vi "Determine More Warnings.vi"(6 "Vitesse max. du vent":dbl, 7 "Vitesse actuelle du vent":dbl, 8 "entrée d'erreur (pas d'erreur)":errorcluster, 9 "Temp. min.":dbl, 10 "Temp. max.":dbl, 11 "Temp. actuelle":dbl) -> (0 "sortie d'erreur":errorcluster, 1 "Mise en garde ?":bool, 2 "Texte de mise en garde":string)   [LabVIEW 2009]
uses:
  Det Warnings.ctl
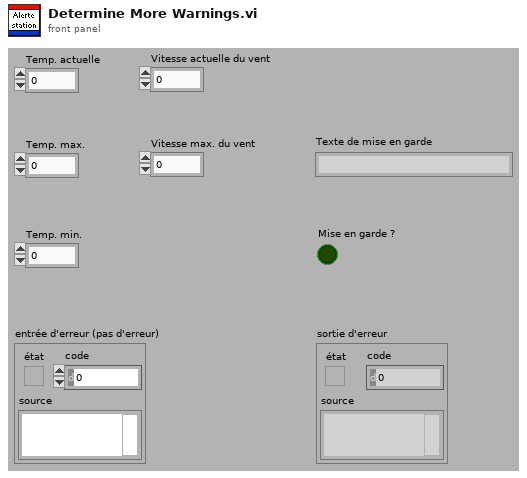
[diagram p1: front panel]
types:
  T1 = typedef "Det Warnings.ctl" = enum16{"Canicule", "Gel", "Vent fort", "Générer une msie en garde", "Détection d'erreur"}
  T2 = cluster{"Temp. actuelle":dbl, "Temp. max.":dbl, "Temp. min.":dbl, "Vitesse actuelle du vent":dbl, "Vitesse max. du vent":dbl}
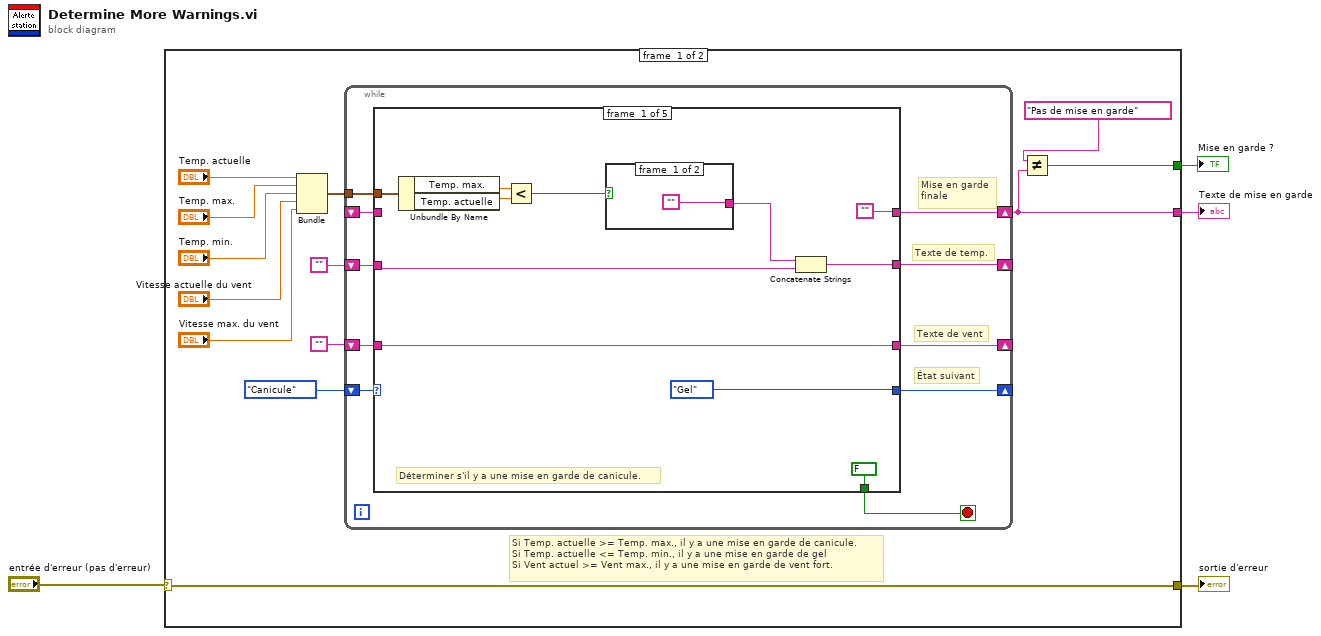
[diagram p0: block diagram]
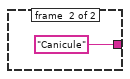
[diagram p2: hidden frame]
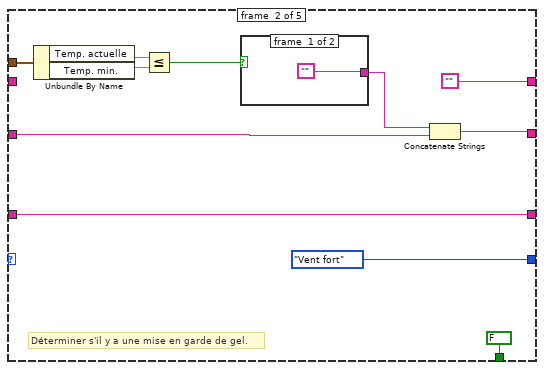
[diagram p3: hidden frame]
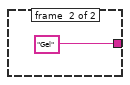
[diagram p4: hidden frame]
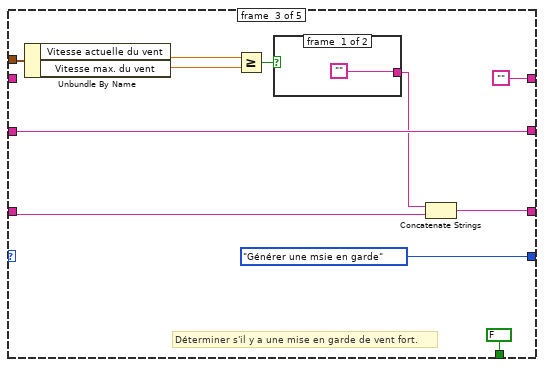
[diagram p5: hidden frame]
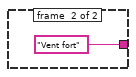
[diagram p6: hidden frame]
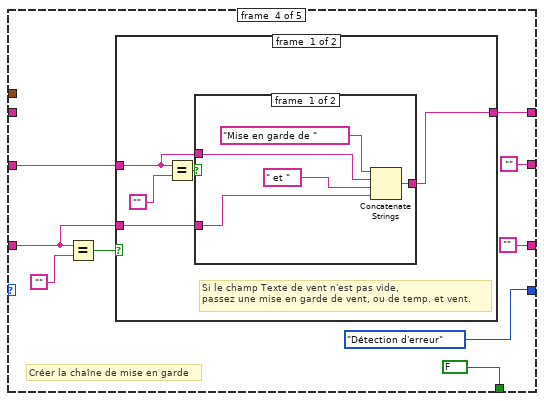
[diagram p7: hidden frame]
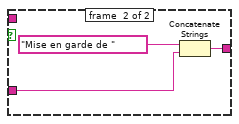
[diagram p8: hidden frame]
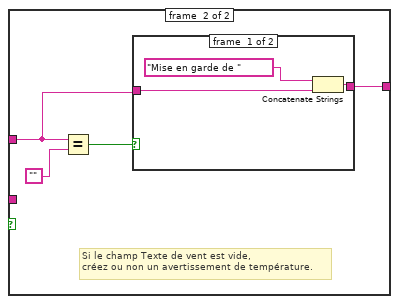
[diagram p9: hidden frame]
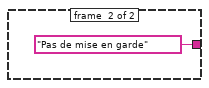
[diagram p10: hidden frame]
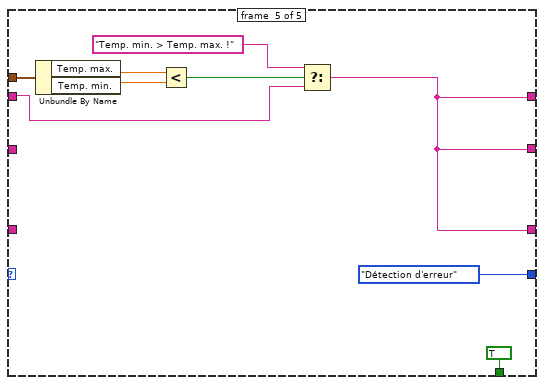
[diagram p11: hidden frame]
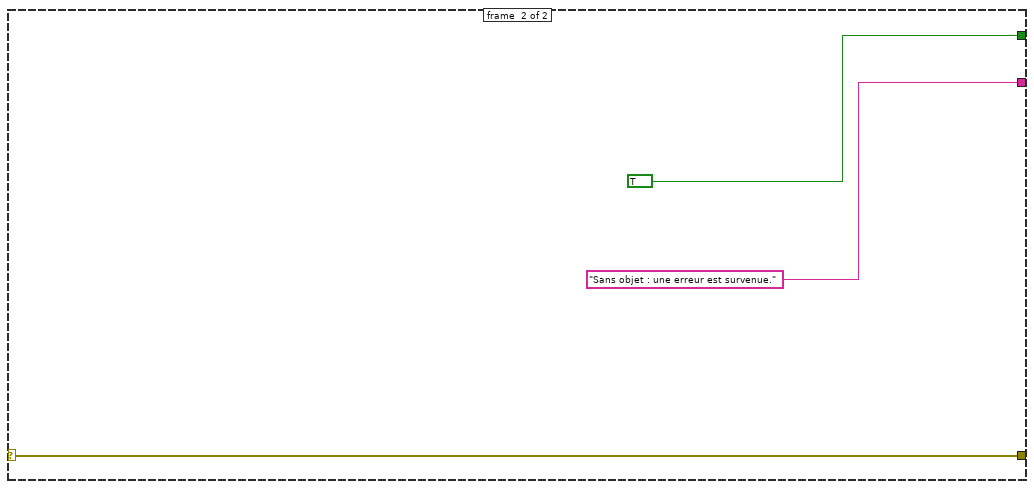
[diagram p12: hidden frame]
diagram:
  n1 = case "Structure Condition" shown="Pas d'erreur" "entrée d'erreur (pas d'erreur)" {
    selector: "entrée d'erreur (pas d'erreur)" -> [w16 w108]
    tunnel: [w16 w108] -> w4
    tunnel: [w17 TRUE] -> w3
    tunnel: [w6 "Sans objet : une erreur est survenue." ("f")] -> w2
    frame #0 {
      # "Si Temp. actuelle >= Temp. max., il y a une mise en garde de canicule.\nSi Temp. actuelle <= Temp. min., il y a une mise en garde de gel\nSi Vent actuel >= Vent max., il y a une mise en garde de vent fort."
      n2 = Bundle ("Assembler")("Temp. actuelle"="Temp. actuelle", "Temp. max."="Temp. max.", "Temp. min."="Temp. min.", "Vitesse actuelle du vent"="Vitesse actuelle du vent", "Vitesse max. du vent"="Vitesse max. du vent") -> (w9:T2)  [unwired: 1 out]
      n3 = while "Boucle While" {
        tunnel: w9 -> [w24]
        shift-right: [w23] -> _
        shift-left: Det_Warnings."Canicule" ("Enum") -> [w27]
        shift-right: [w26] -> _
        shift-left: "" -> [w22]
        shift-right: [w25] -> _
        shift-left: "" -> [w21]
        shift-right: [w20] -> w6
        shift-left: _ -> [w18]
        stop <- w19 stop-if-true
        # "Mise en garde\nfinale"
        # "État suivant"
        # "Texte de vent"
        # "Texte de temp."
        n4 = case shown="\"Canicule\", Par défaut" w27 {
          tunnel: [w30 w46 w58 "" w99] -> w25
          tunnel: [w33 w45 w59 "" w99] -> w26
          tunnel: w24 -> [w37 w51 w64 _ w105]
          tunnel: [Det_Warnings."Gel" ("Enum") Det_Warnings."Vent fort" ("Enum") Det_Warnings."Générer une msie en garde" ("Enum") Det_Warnings."Détection d'erreur" ("Enum") Det_Warnings."Détection d'erreur" ("Enum")] -> w23
          tunnel: w22 -> [w32 w43 w59 w75 _]
          tunnel: w21 -> [w30 w46 w56 w72 _]
          tunnel: ["" "" "" w71 w99] -> w20
          tunnel: [FALSE FALSE FALSE FALSE TRUE] -> w19
          tunnel: w18 -> [_ _ _ _ w101]
          frame #0 {
            # "Déterminer s'il y a une mise en garde de canicule."
            n5 = Unbundle By Name(w37) -> ("Temp. max."=w36:dbl, "Temp. actuelle"=w35:dbl)
            n6 = Less?(x=w36, y=w35) -> (x < y?=w38:bool)
            n7 = case shown="Vrai" w38 {
              tunnel: ["" "Canicule"] -> w31
              frame #0 {
              }
              frame #1 {
              }
            }
            n8 = Concatenate Strings(w31, w32) -> (w33:string)
          }
          frame #1 {
            # "Déterminer s'il y a une mise en garde de gel."
            n9 = Unbundle By Name(w51) -> ("Temp. actuelle"=w49:dbl, "Temp. min."=w48:dbl)
            n10 = Less Or Equal?(x=w49, y=w48) -> (x <= y?=w50:bool)
            n11 = case shown="Vrai" w50 {
              tunnel: ["" "Gel"] -> w44
              frame #0 {
              }
              frame #1 {
              }
            }
            n12 = Concatenate Strings(w44, w43) -> (w45:string)
          }
          frame #2 {
            # "Déterminer s'il y a une mise en garde de vent fort."
            n13 = Unbundle By Name(w64) -> ("Vitesse actuelle du vent"=w63:dbl, "Vitesse max. du vent"=w62:dbl)
            n14 = Greater Or Equal?(x=w63, y=w62) -> (x >= y?=w61:bool)
            n15 = case shown="Vrai" w61 {
              tunnel: ["" "Vent fort"] -> w57
              frame #0 {
              }
              frame #1 {
              }
            }
            n16 = Concatenate Strings(w57, w56) -> (w58:string)
          }
          frame #3 {
            # "Créer la chaîne de mise en garde"
            n17 = Equal?(x=w72, y="") -> (x = y?=w73:bool)
            n18 = case shown="Vrai" w73 {
              tunnel: [w78 w92] -> w71
              tunnel: w75 -> [w76 w89]
              tunnel: w72 -> [w77 _]
              frame #0 {
                # "Si le champ Texte de vent n'est pas vide,\npassez une mise en garde de vent, ou de temp. et vent."
                n19 = Equal?(x=w76, y="") -> (x = y?=w79:bool)
                n20 = case shown="Faux" w79 {
                  tunnel: [w85 w88] -> w78
                  tunnel: w77 -> [w84 w86]
                  tunnel: w76 -> [w82 _]
                  frame #0 {
                    n21 = Concatenate Strings("Mise en garde de " ("string"), w82, " et " ("string"), w84) -> (w85:string)
                  }
                  frame #1 {
                    n22 = Concatenate Strings("Mise en garde de " ("string"), w86) -> (w88:string)
                  }
                }
              }
              frame #1 {
                # "Si le champ Texte de vent est vide, \ncréez ou non un avertissement de température."
                n23 = Equal?(x=w89, y="") -> (x = y?=w90:bool)
                n24 = case shown="Vrai" w90 {
                  tunnel: [w95 "Pas de mise en garde"] -> w92
                  tunnel: w89 -> [w93 _]
                  frame #0 {
                    n25 = Concatenate Strings("Mise en garde de ", w93) -> (w95:string)
                  }
                  frame #1 {
                  }
                }
              }
            }
          }
          frame #4 {
            n26 = Unbundle By Name(w105) -> ("Temp. max."=w104:dbl, "Temp. min."=w103:dbl)
            n27 = Less?(x=w104, y=w103) -> (x < y?=w102:bool)
            n28 = Select(t="Temp. min. > Temp. max. !", s=w102, f=w101) -> (s? t:f=w99:string)
          }
        }
      }
      n29 = Not Equal? ("Différents ?")(x="Pas de mise en garde", y=w6) -> (x != y?=w17:bool)
    }
    frame #1 {
    }
  }
  "sortie d'erreur" <- w4
  "Texte de mise en garde" <- w2
  "Mise en garde ?" <- w3
